vi "Write UUTSupply Event.vi"(8 "error in":errorcluster, 10 "UUTSupply":refnum<user-event>, 11 "Engine in":refnum<class "Engine.lvclass">) -> (0 "error out":errorcluster, 3 "Engine out":refnum<class "Engine.lvclass">)   [LabVIEW 2019, in "Engine.lvlib" / "Engine.lvclass"]
uses:
  Project/Engine.lvclass
  Project/Engine.lvclass/Engine.ctl
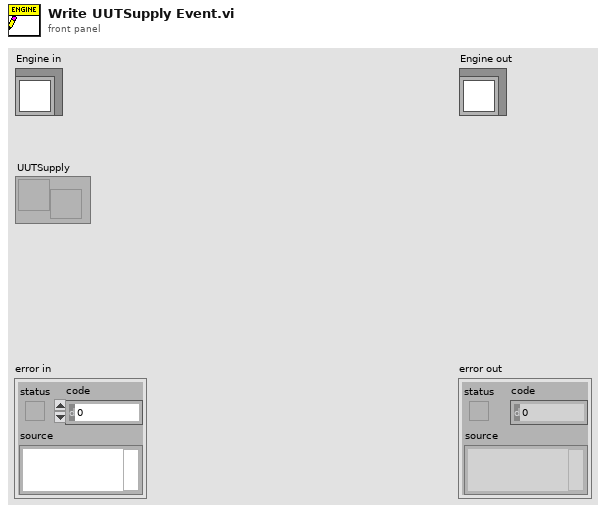
[diagram p1: front panel]
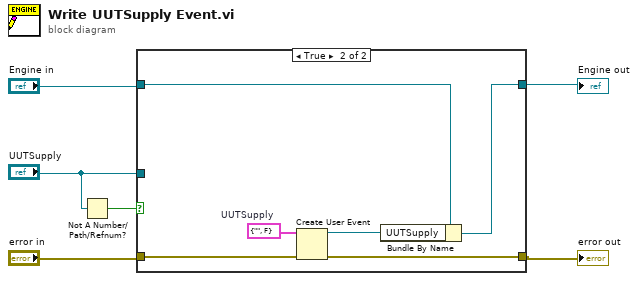
[diagram p0: block diagram]
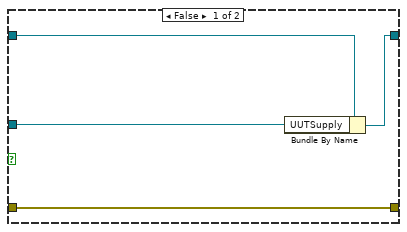
[diagram p2: hidden frame]
diagram:
  n1 = Not A Number/Path/Refnum?(number/path/refnum="UUTSupply") -> (NaN/Path/Refnum?=w4:bool)
  n2 = case shown="True" w4 {
    tunnel: [w7 w14] -> w3
    tunnel: [w9 w13] -> w2
    tunnel: "Engine in" -> [w10 w16]
    tunnel: "UUTSupply" -> [w8 _]
    tunnel: "error in" -> [w7 w15]
    frame False {
      n3 = Bundle By Name(cluster=w10, "UUTSupply"=w8) -> (w9:refnum<class "Engine.lvclass">)
    }
    frame True {
      w12 = cluster{"Supply":string, "Output":bool} {"Supply"="", "Output"=FALSE}  # UUTSupply
      n4 = Create User Event(user event datatype=w12, error in=w15) -> (user event=w11:refnum<user-event>, error out=w14:errorcluster)
      n5 = Bundle By Name(cluster=w16, "UUTSupply"=w11) -> (w13:refnum<class "Engine.lvclass">)
    }
  }
  "error out" <- w3
  "Engine out" <- w2
